vi "Homogenizer.vi"(8 "error in (no error)":errorcluster, 11 "Image in":T1) -> (0 "error out":errorcluster, 3 "Image out":T1)   [LabVIEW 2012]
uses:
  <vilib>/vision/Image Controls.llb/IMAQ Image.ctl
  <vilib>/vision/NI_Vision_Development_Module.lvlib
panel:
  out "System Waveform Graph 2":sgl[](graph)
  out "System Waveform Graph":sgl[](graph)
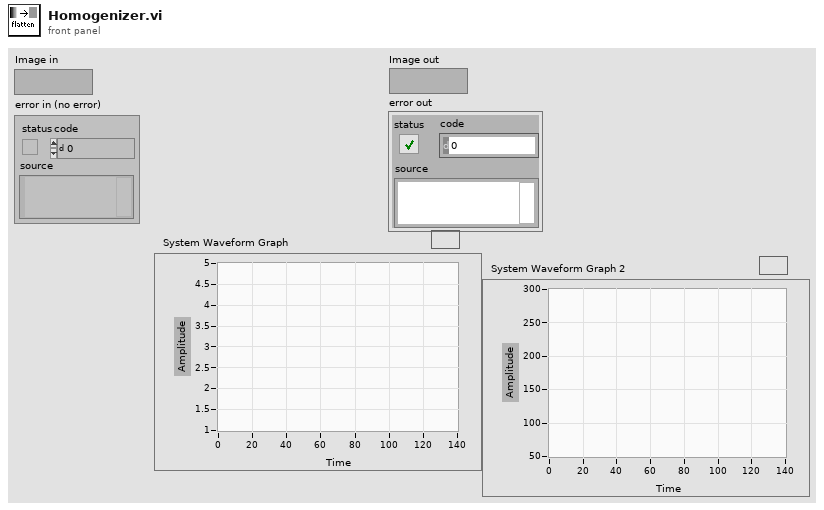
[diagram p1: front panel]
types:
  T1 = typedef "IMAQ Image.ctl" = refnum<image>
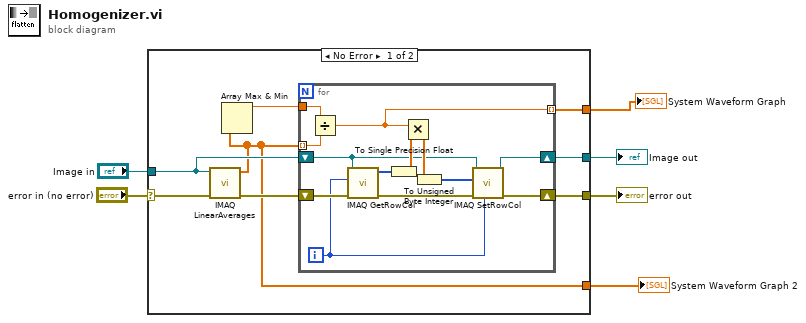
[diagram p0: block diagram]
diagram:
  n1 = case shown="No Error" "error in (no error)" {
    selector: "error in (no error)" -> [w14 w28]
    tunnel: "Image in" -> [w11 w29]
    tunnel: [w10 w29] -> w4
    tunnel: [w9 w28] -> w3
    tunnel: [w8 _] -> w2
    tunnel: [w7 _] -> w1
    frame No Error {
      n2 = call "IMAQ LinearAverages"("error in (no error)"=w14, "Image Src"=w11) -> ("error out"=w12:errorcluster, "Y Axis Averages"=w7:sgl[])  [unwired: 5 in, 3 out]
      n3 = Array Max & Min(array=w7) -> (max value=w13:sgl)  [unwired: 3 out]
      n4 = for {
        tunnel: w7 -> [w26] mode=indexing
        tunnel: w13 -> [w27]
        shift-right: [w19] -> w9
        shift-left: w12 -> [w25]
        shift-right: [w17] -> w10
        shift-left: w11 -> [w18]
        tunnel: [w16] -> w8 mode=indexing
        i -> [w21]
        n5 = Divide(x=w27, y=w26) -> (x/y=w16:sgl)
        n6 = call "IMAQ GetRowCol"("Image"=w18, "Number"=w21, "error in (no error)"=w25) -> ("Pixels (U8)"=w24:u8[], "error out"=w20:errorcluster)  [unwired: 3 in, 3 out]
        n7 = To Single Precision Float(number=w24) -> (single precision float=w22:sgl[])
        n8 = Multiply(x=w16, y=w22) -> (x*y=w23:sgl[])
        n9 = To Unsigned Byte Integer(number=w23) -> (unsigned 8bit integer=w15:u8[])
        n10 = call "IMAQ SetRowCol"("Number"=w21, "error in (no error)"=w20, "Pixels (U8)"=w15, "Image"=w18) -> ("error out"=w19:errorcluster, "Image Out"=w17:T1)  [unwired: 6 in]
      }
    }
    frame Error {
    }
  }
  "Image out" <- w4
  "error out" <- w3
  "System Waveform Graph" <- w2
  "System Waveform Graph 2" <- w1
